vi "Miscellaneous Options.vi"(11 "Full System Configuration":T2={"Rack"=enum."15U; 1-Phase; 16A; 100-240V", "Middle Rail"=enum."None", "Ballast"={"Main"=0, "Small"=0, "Side"=0}, "Front Panel I/O"={"EMO Button"=FALSE, "USB 3.0"=FALSE, "Display"=FALSE, "1st USB 2.0"=FALSE, "2nd USB 2.0"=FALSE, "Ethernet 3"=FALSE, "EMO Extension (3rd Party)"=FALSE, "EMO Extension (Rack In & Out)"=FALSE, "Aux Dual C13 QAC Outlets"=FALSE, "Residual-current Circuit Breaker"=FALSE, "Serial"=FALSE, "GPIB"=FALSE}, "Rear Panel I/O"={"Rear Panel I/O Configuration"=enum."Blank Panel", "EMO Button"=FALSE, "Power, Status & Banana Ground"=FALSE, "Ethernet 2"=FALSE, "Display"=FALSE, "USB 3.0"=FALSE, "DIO"=FALSE, "GPIB"=FALSE, "Aux Dual C13 QAC Outlets"=FALSE, "Residual-current Circuit Breaker"=FALSE, "Serial"=FALSE, "SMA"=FALSE}, "Miscellaneous Options"={"Eyebolts"=FALSE, "Tower Light"=FALSE, "Top/Side Monitor Mount Kit"=FALSE, "24\" Monitor"=FALSE, "Keyboard & Mouse"=FALSE, "Secondary Ethernet Switch"=FALSE, "Extra USB Hub"=FALSE, "USB-6509"=FALSE, "Front Door"=enum."38U (Solid) IG", "Primary Ethernet Switch"=enum."Item 0", "Use Posture"=enum."Item 0"}, "Accessories"={"Screw Type"=enum."10-32", "Cage Nuts & Screws"=0.0, "Filler Panel Color"=enum."Interface Gray", "1U"=0.0, "2U"=0.0, "3U"=0.0}} {"Ballast"."Side" max=5 step=1; "Ballast"."Small" max=5 step=1; "Ballast"."Main" max=5 step=1}) -> (3 "Miscellaneous Options Out":T1[](array[typedef]))   [LabVIEW 2023]
uses:
  Option Type Defs/Full System Configuration.ctl
  Option Type Defs/Rack.ctl
  Option Type Defs/Middle Rail.ctl
  Option Type Defs/Ballast.ctl
  Option Type Defs/Front Panel IO.ctl
  Option Type Defs/Rear Panel IO.ctl
  Option Type Defs/Rear Panel IO Configuration.ctl
  Option Type Defs/Miscellaneous Options.ctl
  Option Type Defs/Front Door.ctl
  Option Type Defs/Accessories.ctl
  Option Type Defs/Screw Types.ctl
  Option Type Defs/Filler Panel Color.ctl
  Option Type Defs/Parts List.ctl
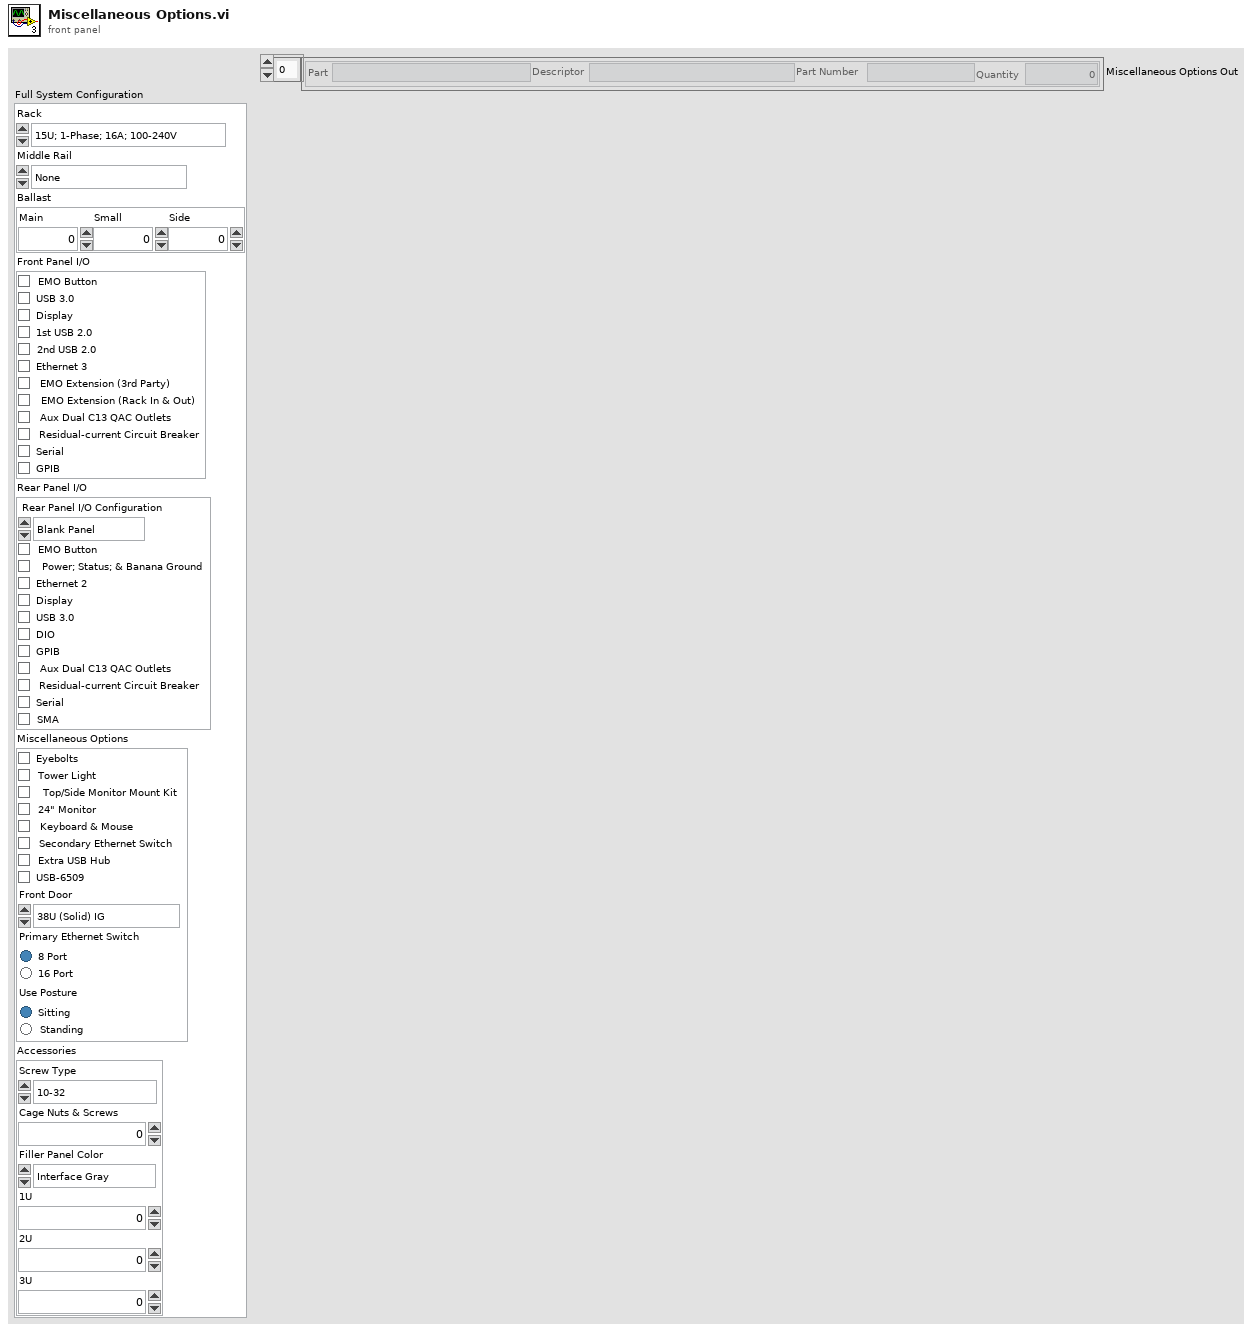
[diagram p1: front panel]
types:
  T1 = typedef "Parts List.ctl" = cluster{"Part":string, "Descriptor":string, "Part Number":string, "Quantity":dbl}
  T2 = typedef "Full System Configuration.ctl" = cluster{"Rack":T3, "Middle Rail":T4, "Ballast":T5, "Front Panel I/O":T6, "Rear Panel I/O":T7, "Miscellaneous Options":T9, "Accessories":T11}
  T3 = typedef "Rack.ctl" = enum16{"15U; 1-Phase; 16A; 100-240V", "15U; 1-Phase; 24A; 100-240V", "38U; 3-Phase Delta; 50A; 200-240V", "38U; 1-Phase; 24A; 100-120V", "38U; 3-Phase Wye; 50A; 200-240V", "38U; 3-Phase Delta; 50A; 380-480V", "38U; 3-Phase Delta; 32A; 200-240V", "38U; 3-Phase Wye; 16A; 100-240V", "44U; 1-Phase; 24A; 100-240V", "44U; 3-Phase Delta; 32A; 200-240V"}
  T4 = typedef "Middle Rail.ctl" = enum16{"None", "Flip Side Rear; D=168.83mm", "Parallel Rear; D=145mm", "Flip Side Front; D=145mm", "Parallel Front; D=145mm"}
  T5 = typedef "Ballast.ctl" = cluster{"Main":u16, "Small":u16, "Side":u16}
  T6 = typedef "Front Panel IO.ctl" = cluster{"EMO Button":bool, "USB 3.0":bool, "Display":bool, "1st USB 2.0":bool, "2nd USB 2.0":bool, "Ethernet 3":bool, "EMO Extension (3rd Party)":bool, "EMO Extension (Rack In & Out)":bool, "Aux Dual C13 QAC Outlets":bool, "Residual-current Circuit Breaker":bool, "Serial":bool, "GPIB":bool}
  T7 = typedef "Rear Panel IO.ctl" = cluster{"Rear Panel I/O Configuration":T8, "EMO Button":bool, "Power, Status & Banana Ground":bool, "Ethernet 2":bool, "Display":bool, "USB 3.0":bool, "DIO":bool, "GPIB":bool, "Aux Dual C13 QAC Outlets":bool, "Residual-current Circuit Breaker":bool, "Serial":bool, "SMA":bool}
  T8 = typedef "Rear Panel IO Configuration.ctl" = enum16{"Blank Panel", "Fully Populated Panel", "Custom Panel"}
  T9 = typedef "Miscellaneous Options.ctl" = cluster{"Eyebolts":bool, "Tower Light":bool, "Top/Side Monitor Mount Kit":bool, "24\" Monitor":bool, "Keyboard & Mouse":bool, "Secondary Ethernet Switch":bool, "Extra USB Hub":bool, "USB-6509":bool, "Front Door":T10, "Primary Ethernet Switch":enum32{"Item 0", "Item 1"}, "Use Posture":enum32{"Item 0", "Item 1"}}
  T10 = typedef "Front Door.ctl" = enum16{"None", "38U (Solid) IG", "38U (Solid) EG", "38U: Top 14U (Solid) IG", "38U (Clear) IG", "44U (Solid) IG", "44U (Solid) EG"}
  T11 = typedef "Accessories.ctl" = cluster{"Screw Type":T12, "Cage Nuts & Screws":dbl, "Filler Panel Color":T13, "1U":dbl, "2U":dbl, "3U":dbl}
  T12 = typedef "Screw Types.ctl" = enum16{"None", "M6 (Most Common)", "10-32", "12-24"}
  T13 = typedef "Filler Panel Color.ctl" = enum16{"None", "Interface Gray", "Environmental Gray"}
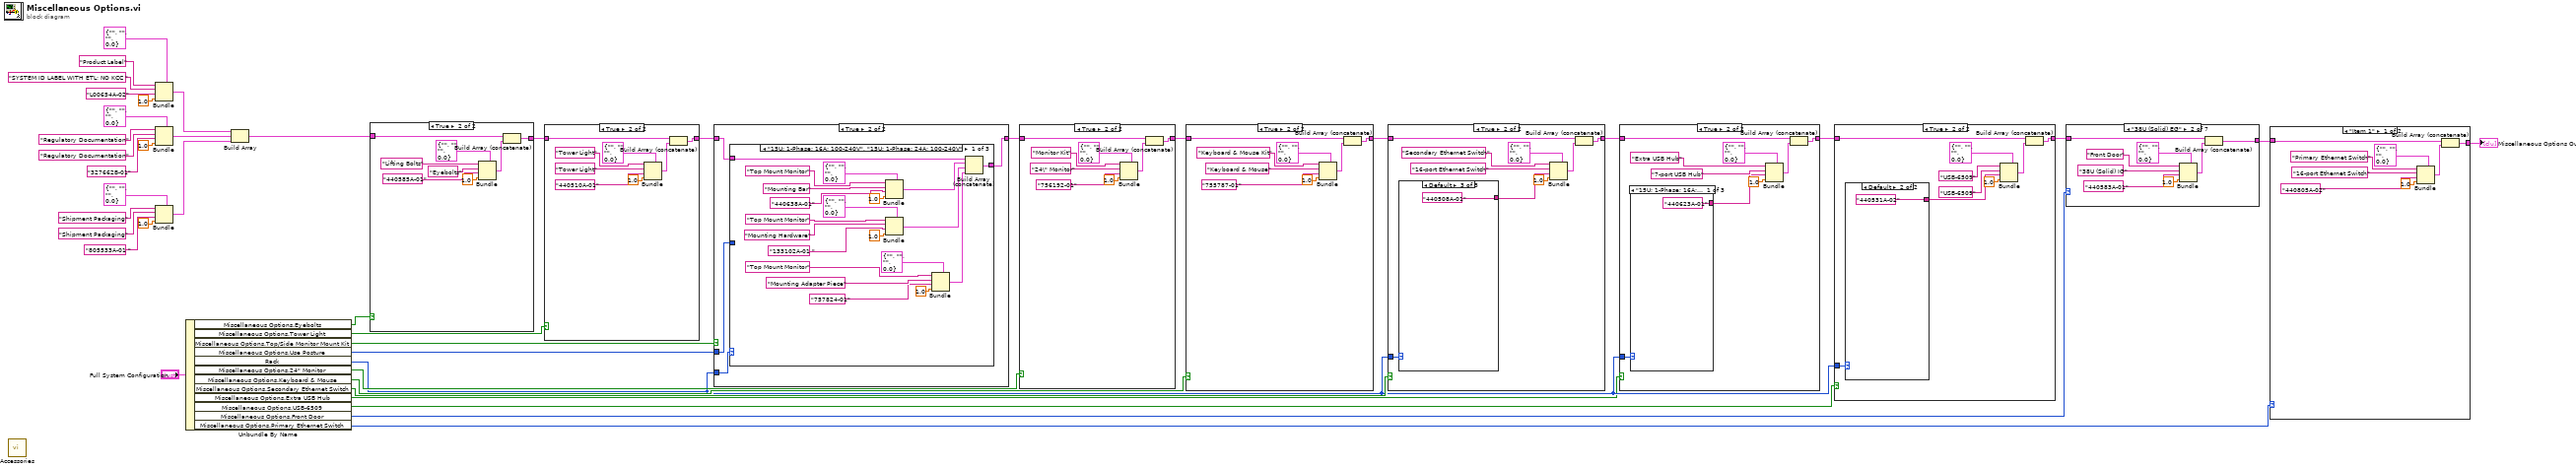
[diagram p0: block diagram]
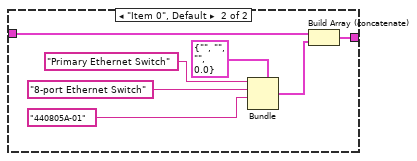
[diagram p2: hidden frame]
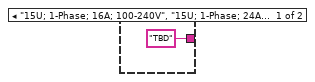
[diagram p4: hidden frame]
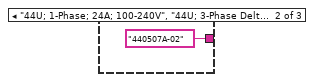
[diagram p6: hidden frame]
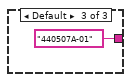
[diagram p7: hidden frame]
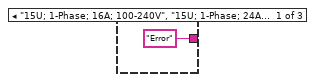
[diagram p9: hidden frame]
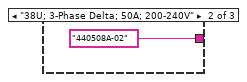
[diagram p10: hidden frame]
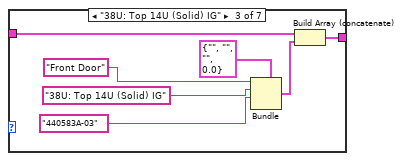
[diagram p14: hidden frame]
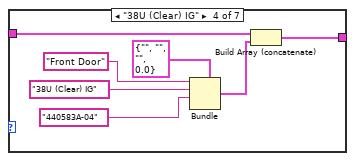
[diagram p15: hidden frame]
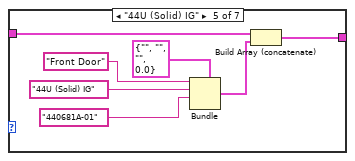
[diagram p16: hidden frame]
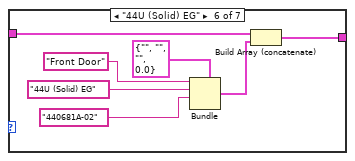
[diagram p17: hidden frame]
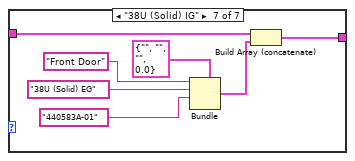
[diagram p18: hidden frame]
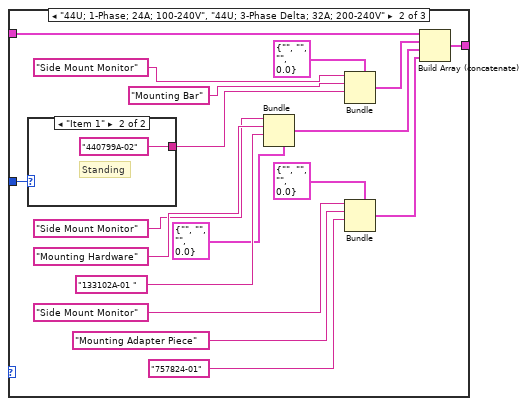
[diagram p20: hidden frame]
diagram:
  n1 = call "Accessories.vi"() -> ()  [unwired: 11 in, 1 out]
  n2 = Bundle(cluster=T1 {"Part"="", "Descriptor"="", "Part Number"="", "Quantity"=0.0}, "Part"="Product Label", "Descriptor"="SYSTEM ID LABEL WITH ETL; NO KCC ", "Part Number"="L00654A-02", "Quantity"=1.0) -> (w38:T1)
  n3 = Bundle(cluster=T1 {"Part"="", "Descriptor"="", "Part Number"="", "Quantity"=0.0}, "Part"="Regulatory Documentation", "Descriptor"="Regulatory Documentation", "Part Number"="327662B-01", "Quantity"=1.0) -> (w33:T1)
  n4 = Bundle(cluster=T1 {"Part"="", "Descriptor"="", "Part Number"="", "Quantity"=0.0}, "Part"="Shipment Packaging", "Descriptor"="Shipment Packaging", "Part Number"="805533A-01 ", "Quantity"=1.0) -> (w28:T1)
  n5 = Unbundle By Name("Full System Configuration") -> ("Miscellaneous Options.Eyebolts"=w26:bool, "Miscellaneous Options.Tower Light"=w24:bool, "Miscellaneous Options.Top/Side Monitor Mount Kit"=w22:bool, "Miscellaneous Options.Use Posture"=w21:enum32{"Item 0", "Item 1"}, "Rack"=w11:T3, "Miscellaneous Options.24\" Monitor"=w18:bool, "Miscellaneous Options.Keyboard & Mouse"=w17:bool, "Miscellaneous Options.Secondary Ethernet Switch"=w15:bool, "Miscellaneous Options.Extra USB Hub"=w8:bool, "Miscellaneous Options.USB-6509"=w4:bool, "Miscellaneous Options.Front Door"=w10:T10, "Miscellaneous Options.Primary Ethernet Switch"=w5:enum32{"Item 0", "Item 1"})
  n6 = Build Array(w38, w33, w28) -> (w27:T1[])
  n7 = case shown="True" w26 {
    tunnel: w27 -> [w43 w51]
    tunnel: [w43 w45] -> w25
    frame False {
    }
    frame True {
      n8 = Bundle(cluster=T1 {"Part"="", "Descriptor"="", "Part Number"="", "Quantity"=0.0}, "Part"="Lifting Bolts", "Descriptor"="Eyebolts", "Part Number"="440585A-01", "Quantity"=1.0) -> (w46:T1)
      n9 = Build Array (concatenate)(w51, w46) -> (w45:T1[])
    }
  }
  n10 = case shown="True" w24 {
    tunnel: w25 -> [w52 w60]
    tunnel: [w52 w54] -> w23
    frame False {
    }
    frame True {
      n11 = Bundle(cluster=T1 {"Part"="", "Descriptor"="", "Part Number"="", "Quantity"=0.0}, "Part"="Tower Light", "Descriptor"="Tower Light", "Part Number"="440510A-01", "Quantity"=1.0) -> (w55:T1)
      n12 = Build Array (concatenate)(w60, w55) -> (w54:T1[])
    }
  }
  n13 = case shown="True" w22 {
    tunnel: w23 -> [w61 w65]
    tunnel: w11 -> [_ w64]
    tunnel: [w61 w62] -> w19
    tunnel: w21 -> [_ w63]
    frame False {
    }
    frame True {
      n14 = case shown="\"15U; 1-Phase; 16A; 100-240V\", \"15U; 1-Phase; 24A; 100-240V\"" w64 {
        tunnel: w65 -> [w85 w103 w123]
        tunnel: [w69 w87 w108] -> w62
        tunnel: w63 -> [_ w86 w107]
        frame "15U; 1-Phase; 16A; 100-240V", "15U; 1-Phase; 24A; 100-240V" {
          n15 = Bundle(cluster=T1 {"Part"="", "Descriptor"="", "Part Number"="", "Quantity"=0.0}, "Part"="Top Mount Monitor", "Descriptor"="Mounting Bar", "Part Number"="440638A-01", "Quantity"=1.0) -> (w80:T1)
          n16 = Bundle(cluster=T1 {"Part"="", "Descriptor"="", "Part Number"="", "Quantity"=0.0}, "Part"="Top Mount Monitor", "Descriptor"="Mounting Hardware", "Part Number"="133102A-01 ", "Quantity"=1.0) -> (w71:T1)
          n17 = Bundle(cluster=T1 {"Part"="", "Descriptor"="", "Part Number"="", "Quantity"=0.0}, "Part"="Top Mount Monitor", "Descriptor"="Mounting Adapter Piece", "Part Number"="757824-01", "Quantity"=1.0) -> (w70:T1)
          n18 = Build Array (concatenate)(w85, w80, w71, w70) -> (w69:T1[])
        }
        frame "44U; 1-Phase; 24A; 100-240V", "44U; 3-Phase Delta; 32A; 200-240V" {
          n19 = case shown="\"Item 1\"" w86 {
            tunnel: ["440799A-01" ("Part Number") "440799A-02" ("Part Number")] -> w99
            frame "Item 0", Default {
              # "Sitting"
            }
            frame "Item 1" {
              # "Standing"
            }
          }
          n20 = Bundle(cluster=T1 {"Part"="", "Descriptor"="", "Part Number"="", "Quantity"=0.0}, "Part"="Side Mount Monitor", "Descriptor"="Mounting Hardware", "Part Number"="133102A-01 ") -> (w89:T1)  [unwired: 1 in]
          n21 = Bundle(cluster=T1 {"Part"="", "Descriptor"="", "Part Number"="", "Quantity"=0.0}, "Part"="Side Mount Monitor", "Descriptor"="Mounting Bar", "Part Number"=w99) -> (w98:T1)  [unwired: 1 in]
          n22 = Bundle(cluster=T1 {"Part"="", "Descriptor"="", "Part Number"="", "Quantity"=0.0}, "Part"="Side Mount Monitor", "Descriptor"="Mounting Adapter Piece", "Part Number"="757824-01") -> (w88:T1)  [unwired: 1 in]
          n23 = Build Array (concatenate)(w103, w98, w89, w88) -> (w87:T1[])
        }
        frame Default {
          n24 = case shown="\"Item 1\"" w107 {
            tunnel: ["440497A-01" ("Part Number") "440497A-02" ("Part Number")] -> w106
            frame "Item 0", Default {
              # "Sitting"
            }
            frame "Item 1" {
              # "Standing"
            }
          }
          n25 = Bundle(cluster=T1 {"Part"="", "Descriptor"="", "Part Number"="", "Quantity"=0.0}, "Part"="Side Mount Monitor", "Descriptor"="Mounting Hardware", "Part Number"="133102A-01 ") -> (w110:T1)  [unwired: 1 in]
          n26 = Bundle(cluster=T1 {"Part"="", "Descriptor"="", "Part Number"="", "Quantity"=0.0}, "Part"="Side Mount Monitor", "Descriptor"="Mounting Bar", "Part Number"=w106) -> (w119:T1)  [unwired: 1 in]
          n27 = Bundle(cluster=T1 {"Part"="", "Descriptor"="", "Part Number"="", "Quantity"=0.0}, "Part"="Side Mount Monitor", "Descriptor"="Mounting Adapter Piece", "Part Number"="757824-01") -> (w109:T1)  [unwired: 1 in]
          n28 = Build Array (concatenate)(w123, w119, w110, w109) -> (w108:T1[])
        }
      }
    }
  }
  n29 = case shown="True" w18 {
    tunnel: w19 -> [w126 w134]
    tunnel: [w126 w128] -> w16
    frame False {
    }
    frame True {
      n30 = Bundle(cluster=T1 {"Part"="", "Descriptor"="", "Part Number"="", "Quantity"=0.0}, "Part"="Monitor Kit", "Descriptor"="24\" Monitor", "Part Number"="756192-01", "Quantity"=1.0) -> (w129:T1)
      n31 = Build Array (concatenate)(w134, w129) -> (w128:T1[])
    }
  }
  n32 = case shown="True" w17 {
    tunnel: w16 -> [w135 w143]
    tunnel: [w135 w137] -> w14
    frame False {
    }
    frame True {
      n33 = Bundle(cluster=T1 {"Part"="", "Descriptor"="", "Part Number"="", "Quantity"=0.0}, "Part"="Keyboard & Mouse Kit", "Descriptor"="Keyboard & Mouse", "Part Number"="755787-01", "Quantity"=1.0) -> (w138:T1)
      n34 = Build Array (concatenate)(w143, w138) -> (w137:T1[])
    }
  }
  n35 = case shown="True" w15 {
    tunnel: w14 -> [w144 w153]
    tunnel: [w144 w147] -> w13
    tunnel: w11 -> [_ w146]
    frame False {
    }
    frame True {
      n36 = case shown="Default" w146 {
        tunnel: ["Error" ("Part Number") "440508A-02" ("Part Number") "440508A-01" ("Part Number")] -> w149
        frame "15U; 1-Phase; 16A; 100-240V", "15U; 1-Phase; 24A; 100-240V" {
        }
        frame "38U; 3-Phase Delta; 50A; 200-240V" {
        }
        frame Default {
        }
      }
      n37 = Bundle(cluster=T1 {"Part"="", "Descriptor"="", "Part Number"="", "Quantity"=0.0}, "Part"="Secondary Ethernet Switch", "Descriptor"="16-port Ethernet Switch", "Part Number"=w149, "Quantity"=1.0) -> (w148:T1)
      n38 = Build Array (concatenate)(w153, w148) -> (w147:T1[])
    }
  }
  n39 = case shown="True" w8 {
    tunnel: w13 -> [w157 w166]
    tunnel: [w157 w160] -> w12
    tunnel: w11 -> [_ w159]
    frame False {
    }
    frame True {
      n40 = case shown="\"15U; 1-Phase; 16A; 100-240V\", \"15U; 1-Phase; 24A; 100-240V\"" w159 {
        tunnel: ["440623A-01" ("Part Number") "440507A-02" ("Part Number") "440507A-01" ("Part Number")] -> w162
        frame "15U; 1-Phase; 16A; 100-240V", "15U; 1-Phase; 24A; 100-240V" {
        }
        frame "44U; 1-Phase; 24A; 100-240V", "44U; 3-Phase Delta; 32A; 200-240V" {
        }
        frame Default {
        }
      }
      n41 = Bundle(cluster=T1 {"Part"="", "Descriptor"="", "Part Number"="", "Quantity"=0.0}, "Part"="Extra USB Hub", "Descriptor"="7-port USB Hub", "Part Number"=w162, "Quantity"=1.0) -> (w161:T1)
      n42 = Build Array (concatenate)(w166, w161) -> (w160:T1[])
    }
  }
  n43 = case shown="True" w4 {
    tunnel: w12 -> [w170 w179]
    tunnel: [w170 w173] -> w9
    tunnel: w11 -> [_ w172]
    frame False {
    }
    frame True {
      n44 = case shown="Default" w172 {
        tunnel: ["TBD" ("Part Number") "440531A-02" ("Part Number")] -> w175
        frame "15U; 1-Phase; 16A; 100-240V", "15U; 1-Phase; 24A; 100-240V" {
        }
        frame Default {
        }
      }
      n45 = Bundle(cluster=T1 {"Part"="", "Descriptor"="", "Part Number"="", "Quantity"=0.0}, "Part"="USB-6509", "Descriptor"="USB-6509", "Part Number"=w175, "Quantity"=1.0) -> (w174:T1)
      n46 = Build Array (concatenate)(w179, w174) -> (w173:T1[])
    }
  }
  n47 = case shown="\"38U (Solid) EG\"" w10 {
    tunnel: w9 -> [w182 w190 w197 w204 w211 w218 w225]
    tunnel: [w182 w184 w191 w198 w205 w212 w219] -> w7
    frame "None", Default {
    }
    frame "38U (Solid) EG" {
      n48 = Bundle(cluster=T1 {"Part"="", "Descriptor"="", "Part Number"="", "Quantity"=0.0}, "Part"="Front Door", "Descriptor"="38U (Solid) IG", "Part Number"="440583A-01", "Quantity"=1.0) -> (w185:T1)
      n49 = Build Array (concatenate)(w190, w185) -> (w184:T1[])
    }
    frame "38U: Top 14U (Solid) IG" {
      n50 = Bundle(cluster=T1 {"Part"="", "Descriptor"="", "Part Number"="", "Quantity"=0.0}, "Part"="Front Door", "Descriptor"="38U: Top 14U (Solid) IG", "Part Number"="440583A-03") -> (w192:T1)  [unwired: 1 in]
      n51 = Build Array (concatenate)(w197, w192) -> (w191:T1[])
    }
    frame "38U (Clear) IG" {
      n52 = Bundle(cluster=T1 {"Part"="", "Descriptor"="", "Part Number"="", "Quantity"=0.0}, "Part"="Front Door", "Descriptor"="38U (Clear) IG", "Part Number"="440583A-04") -> (w199:T1)  [unwired: 1 in]
      n53 = Build Array (concatenate)(w204, w199) -> (w198:T1[])
    }
    frame "44U (Solid) IG" {
      n54 = Bundle(cluster=T1 {"Part"="", "Descriptor"="", "Part Number"="", "Quantity"=0.0}, "Part"="Front Door", "Descriptor"="44U (Solid) IG", "Part Number"="440681A-01") -> (w206:T1)  [unwired: 1 in]
      n55 = Build Array (concatenate)(w211, w206) -> (w205:T1[])
    }
    frame "44U (Solid) EG" {
      n56 = Bundle(cluster=T1 {"Part"="", "Descriptor"="", "Part Number"="", "Quantity"=0.0}, "Part"="Front Door", "Descriptor"="44U (Solid) EG", "Part Number"="440681A-02") -> (w213:T1)  [unwired: 1 in]
      n57 = Build Array (concatenate)(w218, w213) -> (w212:T1[])
    }
    frame "38U (Solid) IG" {
      n58 = Bundle(cluster=T1 {"Part"="", "Descriptor"="", "Part Number"="", "Quantity"=0.0}, "Part"="Front Door", "Descriptor"="38U (Solid) EG", "Part Number"="440583A-01") -> (w220:T1)  [unwired: 1 in]
      n59 = Build Array (concatenate)(w225, w220) -> (w219:T1[])
    }
  }
  n60 = case shown="\"Item 1\"" w5 {
    tunnel: w7 -> [w233 w240]
    tunnel: [w227 w234] -> w6
    frame "Item 1" {
      n61 = Bundle(cluster=T1 {"Part"="", "Descriptor"="", "Part Number"="", "Quantity"=0.0}, "Part"="Primary Ethernet Switch", "Descriptor"="16-port Ethernet Switch", "Part Number"="440805A-02", "Quantity"=1.0) -> (w228:T1)
      n62 = Build Array (concatenate)(w233, w228) -> (w227:T1[])
    }
    frame "Item 0", Default {
      n63 = Bundle(cluster=T1 {"Part"="", "Descriptor"="", "Part Number"="", "Quantity"=0.0}, "Part"="Primary Ethernet Switch", "Descriptor"="8-port Ethernet Switch", "Part Number"="440805A-01") -> (w235:T1)  [unwired: 1 in]
      n64 = Build Array (concatenate)(w240, w235) -> (w234:T1[])
    }
  }
  "Miscellaneous Options Out" <- w6
